vi "Read_protocols_file_and_init_array_of_protocols.vi"(8 "error in (no error)":errorcluster, 10 "Comm master cluster":T1={"Main event var"=refnum, "VIRef"=refnum, "Data path"=path "", "Reads"=0, "total number of UUT"=0, "FF refnum"={"Handle1"=0, "Handle2"=0}, "FF device id list"=[], "MODBUS resource name"="", "MODBUS Serial Parameters"={"Mode"=enum."RTU", "Default Slave Address"=0, "MODBUS timeout"=0, "Baud Rate"=0, "Parity"=0, "Flow Control"=0}, "Profibus resource name"="", "Profibus Communication ref.:"=0, "HART resource name"="", "HART long addresses (array)"=[], "Comm relay session"="", "Comm UI event"=refnum, "Write Interval (s)"=5.0, "DMM_QUEUE"=refnum, "POWER_QUEUE"=refnum, "\nTHERM_QUEUE"=refnum, "\nCOMM_QUEUE"=refnum, "TIMING_QUEUE"=refnum, "MAIN_QUEUE"=refnum, "Log path"=path ""} {"Write Interval (s)" min=0.1 max=1000.0 step=0.1}, 11 "Protocol in":refnum<class "Protocol.lvclass">) -> (0 "error out":errorcluster, 1 "Array of configured protocols":string[](array[string]), 2 "Array of Protocols out":refnum<class "Protocol.lvclass">[](array[class]), 3 "Protocol out":refnum<class "Protocol.lvclass">)   [LabVIEW 2016, in "Protocol.lvclass"]
uses:
  Protocol.lvclass
  MASTER_OPC.ctl
  Typedef/event var.ctl
  Typedef/Comm ui action type.ctl
  Typedef/Comm_State_enum.ctl
  Typedef/state var.ctl
  Typedef/Protocol_enum_type.ctl
  MODBUS/MODBUS Class/MODBUS.lvclass
  C:/Users/d/Desktop/Software/Micromotion/Mark Lee/Source (1.09 US LV 2016)/Blackbox/OPC Server/Protocol Class/Protocol.lvclass
  HART/HART Class/HART.lvclass
  DeviceNET/DeviceNET Class/DeviceNET.lvclass
  Protocol.lvclass/Protocol.ctl
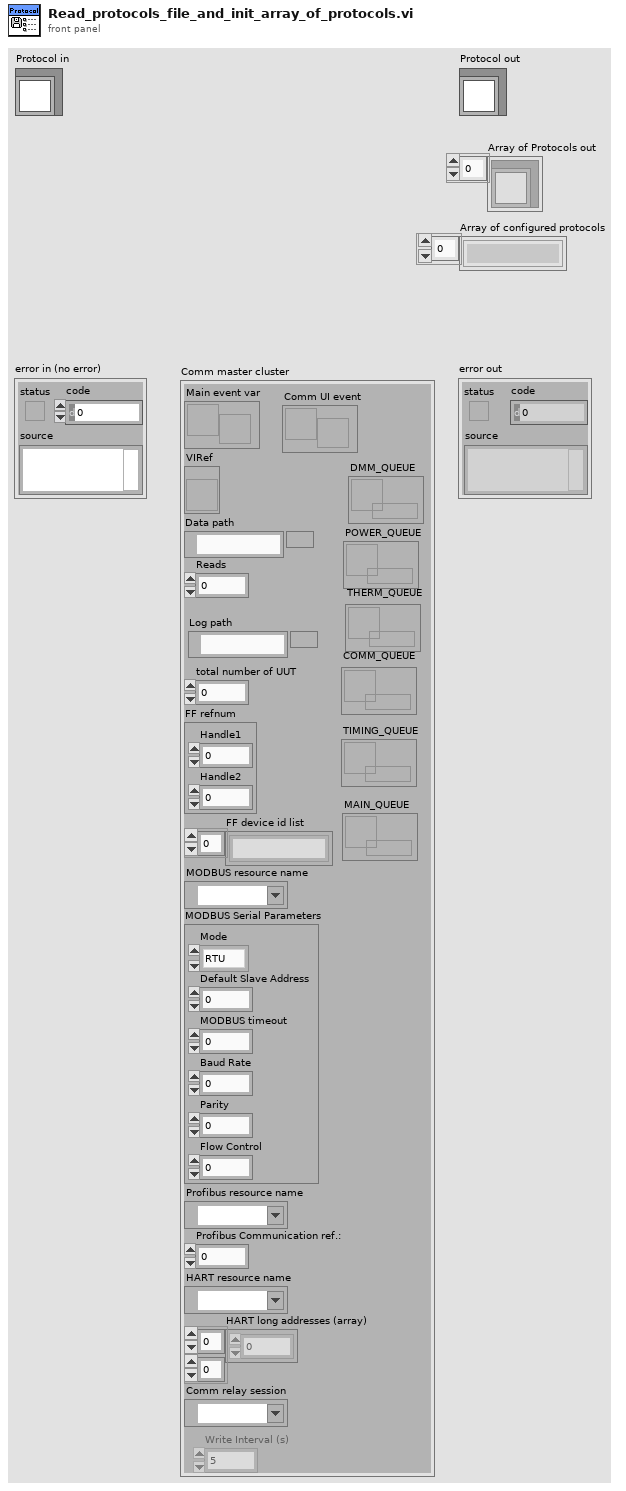
[diagram p1: front panel]
types:
  T1 = typedef "MASTER_OPC.ctl" = cluster{"Main event var":refnum<user-event>, "VIRef":refnum<vi>, "Data path":path, "Reads":i32, "total number of UUT":i32, "FF refnum":cluster{"Handle1":u32, "Handle2":u32}, "FF device id list":string[], "MODBUS resource name":refnum<visa-resource-name>, "MODBUS Serial Parameters":cluster{"Mode":enum16{"RTU", "ASCII"}, "Default Slave Address":u8, "MODBUS timeout":u32, "Baud Rate":u32, "Parity":u16, "Flow Control":u16}, "Profibus resource name":refnum<visa-resource-name>, "Profibus Communication ref.:":u8, "HART resource name":refnum<visa-resource-name>, "HART long addresses (array)":u8[][], "Comm relay session":refnum<k15>, "Comm UI event":refnum<user-event>, "Write Interval (s)":dbl, "DMM_QUEUE":refnum<queue>, "POWER_QUEUE":refnum<queue>, "\nTHERM_QUEUE":refnum<queue>, "\nCOMM_QUEUE":refnum<queue>, "TIMING_QUEUE":refnum<queue>, "MAIN_QUEUE":refnum<queue>, "Log path":path}
  T2 = typedef "Protocol_enum_type.ctl" = enum16{"None", "MODBUS", "HART", "Fieldbus", "Profibus DP", "Profibus PA", "DeviceNET", "USB"}
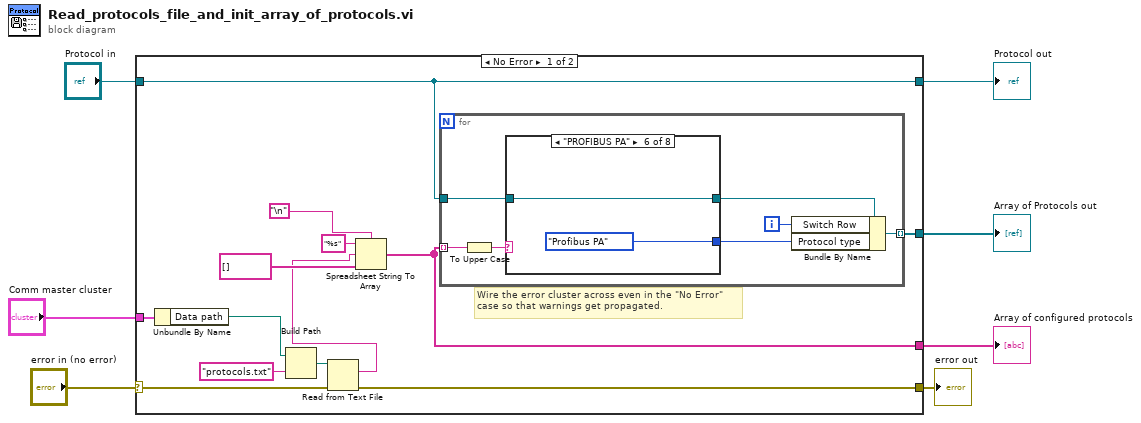
[diagram p0: block diagram]
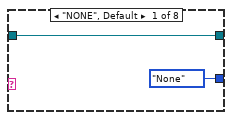
[diagram p2: hidden frame]
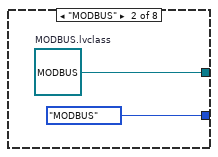
[diagram p3: hidden frame]
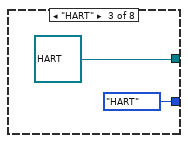
[diagram p4: hidden frame]
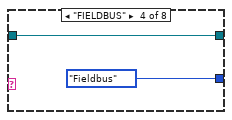
[diagram p5: hidden frame]
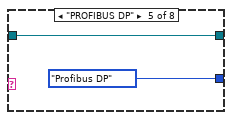
[diagram p6: hidden frame]
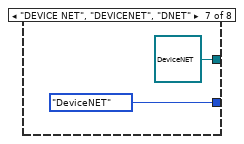
[diagram p7: hidden frame]
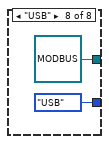
[diagram p8: hidden frame]
diagram:
  n1 = case shown="No Error" "error in (no error)" {
    selector: "error in (no error)" -> [w13 w45]
    tunnel: [w14 w45] -> w6
    tunnel: [w16 w44] -> w4
    tunnel: "Protocol in" -> [w16 w44]
    tunnel: "Comm master cluster" -> [w17 _]
    tunnel: [w15 _] -> w2
    tunnel: [w9 _] -> w1
    frame No Error {
      # "Wire the error cluster across even in the \"No Error\"\ncase so that warnings get propagated."
      n2 = Unbundle By Name(w17) -> ("Data path"=w18:path)
      n3 = Build Path(base path=w18, name or relative path="protocols.txt") -> (appended path=w19:path)
      n4 = Read from Text File(file (use dialog)=w19, error in=w13) -> (text=w10:string, error out=w14:errorcluster)  [unwired: 2 in, 2 out]
      n5 = Spreadsheet String To Array(delimiter (Tab)="\n", format string="%s", spreadsheet string=w10, array type (2D Dbl)=string[] [] ("Array of Strings")) -> (array=w9:string[])
      n6 = for {
        tunnel: w9 -> [w24] mode=indexing
        tunnel: w16 -> [w21]
        tunnel: [w26] -> w15 mode=indexing
        i -> [w27]
        n7 = To Upper Case(1:w24) -> (0:w25:string)
        n8 = case shown="\"PROFIBUS PA\"" w25 {
          tunnel: [Protocol_enum_type."None" ("Protocol type") Protocol_enum_type."MODBUS" ("Protocol type") Protocol_enum_type."HART" ("Protocol type") Protocol_enum_type."Fieldbus" ("Protocol type") Protocol_enum_type."Profibus DP" ("Protocol type") Protocol_enum_type."Profibus PA" ("Protocol type") Protocol_enum_type."DeviceNET" ("Protocol type") Protocol_enum_type."USB" ("Protocol type")] -> w23
          tunnel: [w28 w30 refnum<class "HART.lvclass"> refnum ("HART.lvclass") w34 w36 w38 refnum<class "DeviceNET.lvclass"> refnum ("DeviceNET.lvclass") refnum<class "MODBUS.lvclass"> refnum ("MODBUS.lvclass")] -> w22
          tunnel: w21 -> [w28 _ _ w34 w36 w38 _ _]
          frame "NONE", Default {
          }
          frame "MODBUS" {
            w30 = refnum<class "MODBUS.lvclass"> refnum  # MODBUS.lvclass
          }
          frame "HART" {
          }
          frame "FIELDBUS" {
          }
          frame "PROFIBUS DP" {
          }
          frame "PROFIBUS PA" {
          }
          frame "DEVICE NET", "DEVICENET", "DNET" {
          }
          frame "USB" {
          }
        }
        n9 = Bundle By Name(cluster=w22, "Switch Row"=w27, "Protocol type"=w23) -> (w26:refnum<class "Protocol.lvclass">)
      }
    }
    frame Error {
    }
  }
  "error out" <- w6
  "Protocol out" <- w4
  "Array of Protocols out" <- w2
  "Array of configured protocols" <- w1
